vi "Build Report.vi"(8 "error in (no error)":errorcluster, 9 "Report Data":T4[](array[typedef]), 10 "Steps":T1[](array[typedef]), 11 "Path":path) -> (0 "error out":errorcluster)   [LabVIEW 2020, in "MacroAssert.lvlib"]
uses:
  MacroAssert.lvlib
  CTLs/Step Type V3.ctl
  CTLs/Assertion Type.ctl
  CTLs/Step V3.ctl
  CTLs/Report Data.ctl
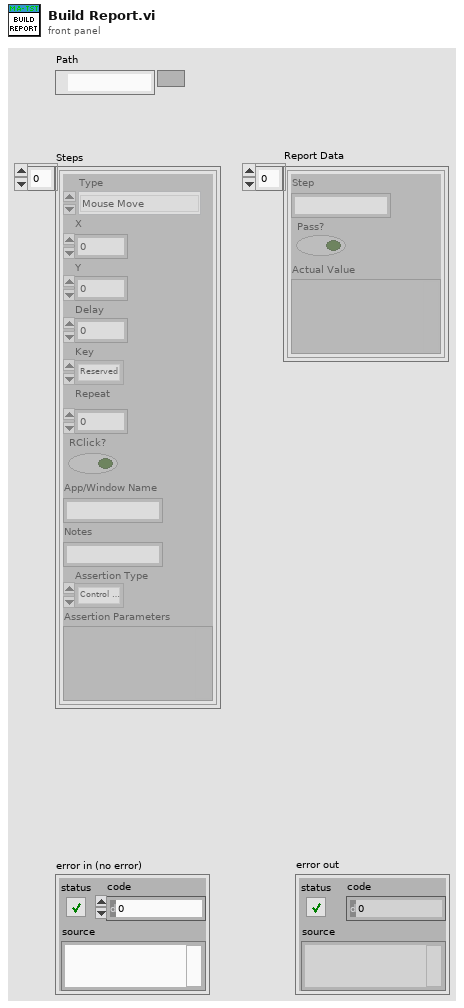
[diagram p1: front panel]
types:
  T1 = typedef "MacroAssert.lvlib/Step V3.ctl" = cluster{"Type":T2, "X":i32, "Y":i32, "Delay":i32, "Key":u8, "Repeat":i32, "RClick?":bool, "App/Window Name":string, "Notes":string, "Assertion Type":T3, "Assertion Parameters":variant}
  T2 = typedef "MacroAssert.lvlib/Step Type V3.ctl" = enum16{"Mouse Move", "Mouse Click", "Key Press", "Wait", "Mouse Down", "Mouse Up", "Key Down", "Key Up", "Test Assertion", "Run Application", "Maximize Window", "Restore Window", "Minimize Window", "Close Window", "Bring Window to Front", "Send Window to Back"}
  T3 = typedef "MacroAssert.lvlib/Assertion Type.ctl" = enum16{"Control Position", "Control Visible", "Control Disabled", "Control Image"}
  T4 = typedef "MacroAssert.lvlib/Report Data.ctl" = cluster{"Step":string, "Pass?":bool, "Actual Value":variant}
  T5 = enum16{"open", "replace", "create", "open or create", "replace or create", "replace or create with confirmation"}
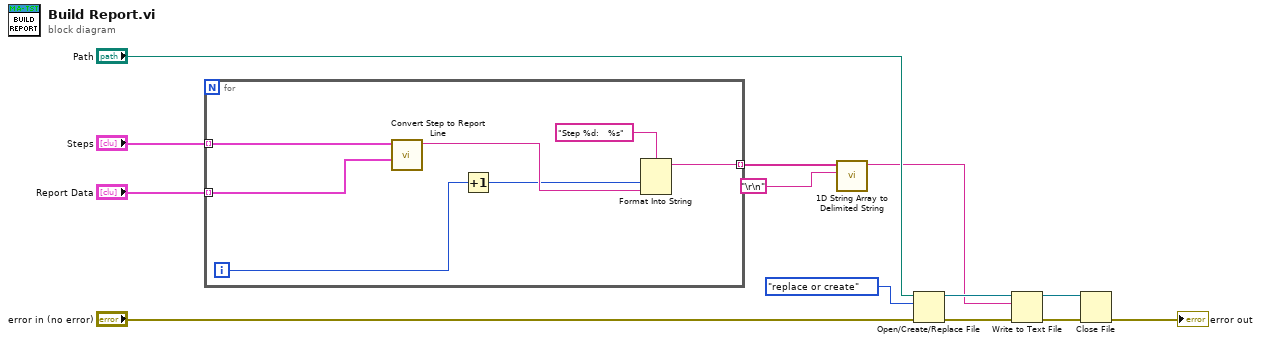
[diagram p0: block diagram]
diagram:
  n1 = for {
    tunnel: "Steps" -> [w20] mode=indexing
    tunnel: "Report Data" -> [w19] mode=indexing
    tunnel: [w14] -> w3 mode=indexing
    i -> [w16]
    n2 = call "Convert Step to Report Line.vi"("Report Data"=w19, "Step"=w20) -> ("Report Line"=w17:string)  [unwired: 9 in]
    n3 = Increment(x=w16) -> (x+1=w15:i32)
    n4 = Format Into String(format string="Step %d:   %s", w15, w17) -> (resulting string=w14:string)  [unwired: 2 in, 1 out]
  }
  n5 = call <vilib>:"1D String Array to Delimited String.vi"("delimiter"="\r\n", "string array"=w3) -> ("delimited string"=w2:string)  [unwired: 9 in]
  n6 = Open/Create/Replace File(file path (use dialog)="Path", error in="error in (no error)", operation (0:open)=T5."replace or create") -> (refnum out=w11:refnum<file>, error out=w10:errorcluster)  [unwired: 3 in, 1 out]
  n7 = Write to Text File(file (use dialog)=w11, text=w2, error in=w10) -> (refnum out=w9:refnum<file>, error out=w8:errorcluster)  [unwired: 1 in, 1 out]
  n8 = Close File(refnum=w9, error in=w8) -> (error out=→"error out":errorcluster)  [unwired: 1 out]
